vi "DFD FXP C Code Generator.vi"(6 "confirm? (T)":bool=TRUE, 8 "error in (no error)":errorcluster, 9 "filter name":string, 10 "destination folder":path, 11 "filter in":T1={"mSRate_Fs"=1.0, "mSRate_Version"="2.0", "mSRate_Comments"="", "mSRate_OrgCoef"={"type"=enum."Undefined", "gain"=1.0, "coef a (k)"=[], "coef b (v)"=[]}, "mSRate_CurCoef"={"type"=enum."Undefined", "gain"=1.0, "coef a (k)"=[], "coef b (v)"=[]}, "mSRate_Quantized?"=FALSE, "mSRate_QCoef"={"type"=enum."Undefined", "gain"=1.0, "coef a (k)"=[], "coef b (v)"=[]}, "mSRate_QSettings"=[], "mSRate_Order"=0, "mSRate_Scaling"={"mSRate_ScaleByPowerOf2?"=FALSE, "mSRate_ScaleType"=enum."No Norm"}} {"mSRate_QSettings"."source" items=["Coef a/k"=0, "Coef b/v"=7, "Input"=1, "Output"=2, "Multiplicand"=3, "Product"=4, "Sum"=5, "Delay"=6, "Gain"=8]}) -> (0 "error out":errorcluster, 2 "output files":path[](array[path]))   [LabVIEW 2017, in "NI_DigFilterLicensed.lvlib"]
doc: "Generates fixed-point code from a fixed-point filter, including fixed-point LabVIEW field-programmable gate array (FPGA) code, integer LabVIEW code, and C code. You must manually select the polymorphic instance you want to use."
uses:
  <vilib>/addons/Digital Filter Design/NI_DigFilterLicensed.lvlib
  <vilib>/addons/Digital Filter Design/_Objects.llb/DFD Filter Obj.ctl
  <vilib>/addons/Digital Filter Design/_Objects.llb/DFD Filter Coef.ctl
  <vilib>/addons/Digital Filter Design/_Objects.llb/DFD Filter Structure Type Selector.ctl
  <vilib>/addons/Digital Filter Design/_Objects.llb/dfd_Internal Quantization Settings.ctl
  <vilib>/addons/Digital Filter Design/_Objects.llb/dfd_Internal Quantization Srcs.ctl
  <vilib>/addons/Digital Filter Design/_Objects.llb/DFD Coef Norm Type.ctl
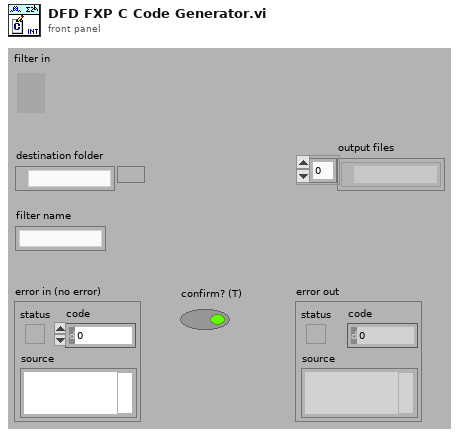
[diagram p1: front panel]
types:
  T1 = typedef "NI_DigFilterLicensed.lvlib/DFD Filter Obj.ctl" = cluster{"mSRate_Fs":dbl, "mSRate_Version":string, "mSRate_Comments":string, "mSRate_OrgCoef":T2, "mSRate_CurCoef":T2, "mSRate_Quantized?":bool, "mSRate_QCoef":T2, "mSRate_QSettings":T4[], "mSRate_Order":i32, "mSRate_Scaling":cluster{"mSRate_ScaleByPowerOf2?":bool, "mSRate_ScaleType":T6}}
  T2 = typedef "NI_DigFilterLicensed.lvlib/DFD Filter Coef.ctl" = cluster{"type":T3, "gain":dbl, "coef a (k)":dbl[], "coef b (v)":dbl[]}
  T3 = typedef "NI_DigFilterLicensed.lvlib/DFD Filter Structure Type Selector.ctl" = enum16{"Undefined", "FIR Direct Form", "FIR Direct Form Transposed", "FIR Symmetric", "FIR Antisymmetric", "IIR Direct Form I", "IIR Direct Form I Transposed", "IIR Direct Form II", "IIR Direct Form II Transposed", "IIR Cascaded Second Order Sections Form I", "IIR Cascaded Second Order Sections Form I Transposed", "IIR Cascaded Second Order Sections Form II", "IIR Cascaded Second Order Sections Form II Transposed", "Lattice Allpass (basic sections)", "Lattice Allpass (one multiplier sections)", "Lattice Allpass (normalized sections)", "Lattice AR (basic sections)", "Lattice AR (one multiplier sections)", "Lattice AR (normalized sections)", "Lattice MA (minimum phase)", "Lattice MA (maximum phase)", "Lattice ARMA (basic sections)", "Lattice ARMA (one multiplier sections)", "Lattice ARMA (normalized sections)"}
  T4 = typedef "NI_DigFilterLicensed.lvlib/dfd_Internal Quantization Settings.ctl" = cluster{"source":T5, "wl":i16, "iwl":i16, "overflow mode":enum16{"Saturation", "Wrap"}, "rounding mode":enum16{"Nearest", "Truncation"}, "signed?":bool}
  T5 = typedef "NI_DigFilterLicensed.lvlib/dfd_Internal Quantization Srcs.ctl" = u16
  T6 = typedef "NI_DigFilterLicensed.lvlib/DFD Coef Norm Type.ctl" = enum16{"No Norm", "Time Domain 1-Norm", "Time Domain 2-Norm", "Time Domain Inf-Norm"}
  T7 = cluster{"C":refnum<file>, "H":refnum<file>, "typedef":refnum<file>}
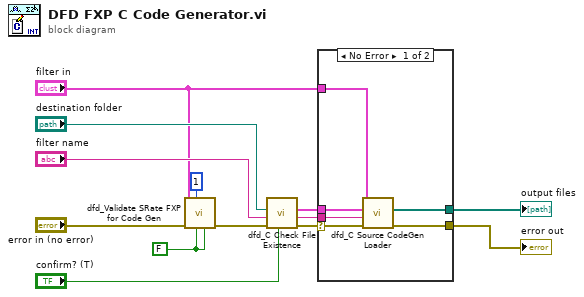
[diagram p0: block diagram]
diagram:
  w5 = FALSE ("LabVIEW?")
  n1 = call <vilib>:"dfd_Validate SRate FXP for Code Gen.vi"("FPGA?"=w5, "LabVIEW?"=w5, "totalChan"=1, "error in"="error in (no error)", "filter"="filter in") -> ("error out"=w2:errorcluster)  [unwired: 6 out]
  n2 = call <vilib>:"dfd_C Check File Existence.vi"("confirm?"="confirm? (T)", "error in (no error)"=w2, "filter name"="filter name", "dest path"="destination folder") -> ("error out"=w1:errorcluster, "filter name out"=w9:string, "dest file refs"=w8:T7)  [unwired: 5 out]
  n3 = case shown="No Error" w1 {
    selector: w1 -> [w19 w20]
    tunnel: "filter in" -> [w14 _]
    tunnel: w9 -> [w18 _]
    tunnel: w8 -> [w17 _]
    tunnel: [w16 _] -> w7
    tunnel: [w15 w20] -> w6
    frame No Error {
      n4 = call <vilib>:"dfd_C Source CodeGen Loader.vi"("error in (no error)"=w19, "filter name"=w18, "dest file refs"=w17, "filter in"=w14) -> ("error out"=w15:errorcluster, "output files"=w16:path[])  [unwired: 6 out]
    }
    frame Error {
    }
  }
  "error out" <- w6
  "output files" <- w7
